vi "MSEncoder Case-4-IonGate.vi"(8 "error in (no error)":errorcluster, 9 "ParamValIn":variant, 11 "MSEncoder in":refnum<class "MSEncoder.lvclass">) -> (0 "error out":errorcluster, 3 "MSEncoder out":refnum<class "MSEncoder.lvclass">)   [LabVIEW 2018, in "MSEncoder.lvclass"]
uses:
  MSEncoder.lvclass
  Ctl/MSEditorParam ionGate.ctl
  MSEncoder.lvclass/MSEncoder.ctl
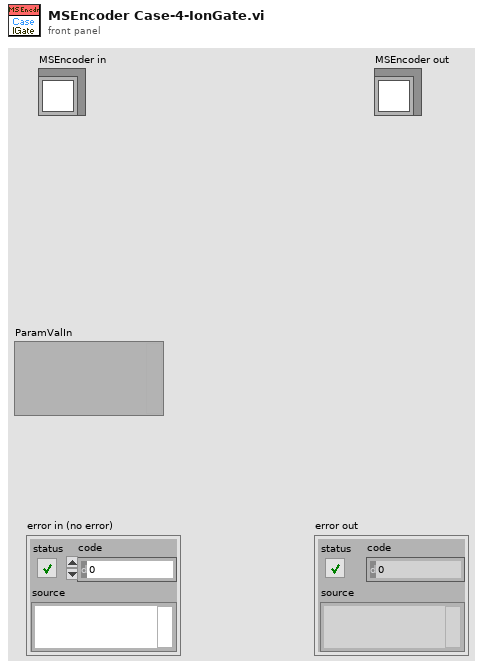
[diagram p1: front panel]
types:
  T1 = typedef "MSEditorParam ionGate.ctl" = cluster{"trialTime":ext, "TPH":ext, "enableAGC":bool}
  T2 = cluster{"Label":string, "dt":dbl, "Length":u32, "RefVolt":dbl, "mzTable":cluster{"t":dbl[], "mz":dbl[], "beta":dbl[]}}[]
  T3 = cluster{"Label":string, "dt":dbl, "Length":u32, "RefVolt":dbl, "mzTable":cluster{"t":dbl[], "mz":dbl[], "beta":dbl[]}}
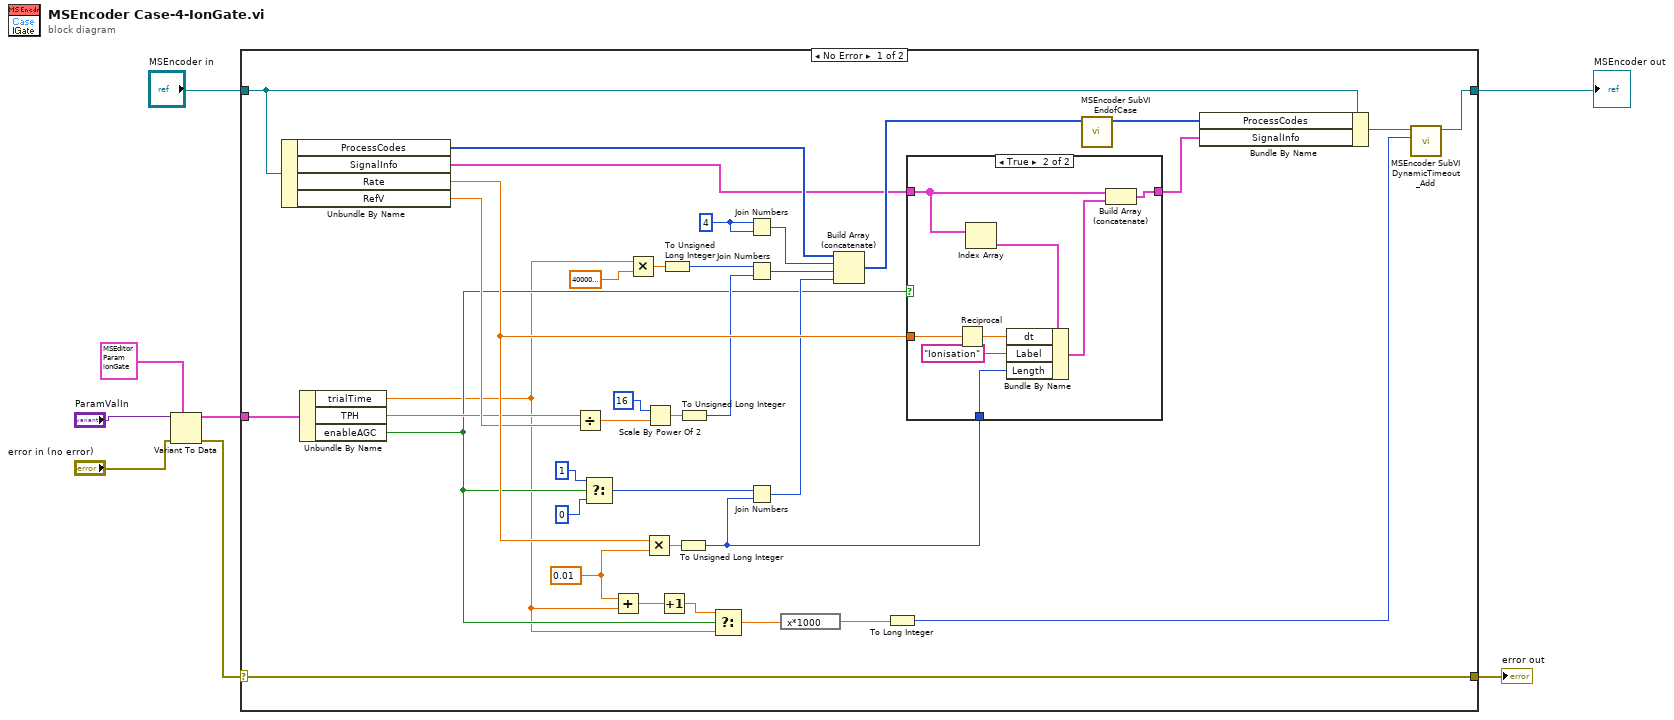
[diagram p0: block diagram]
diagram:
  n1 = Variant To Data(error in="error in (no error)", type=T1 {"trialTime"=0.1, "TPH"=1.0, "enableAGC"=FALSE} ("ParamValueType"), Variant="ParamValIn") -> (data=w2:T1, error out=w1:errorcluster)
  n2 = case shown="No Error" w1 {
    selector: w1 -> [w44 w56]
    tunnel: "MSEncoder in" -> [w43 w55]
    tunnel: [w44 w56] -> w8
    tunnel: [w17 w55] -> w6
    tunnel: w2 -> [w20 _]
    frame No Error {
      w11 = 0.01 ("y")
      w36 = u32 4
      n3 = Unbundle By Name(w43) -> ("ProcessCodes"=w45:u64[], "SignalInfo"=w15:T2, "Rate"=w41:dbl, "RefV"=w39:dbl)
      n4 = Unbundle By Name(w20) -> ("trialTime"=w10:ext, "TPH"=w21:ext, "enableAGC"=w16:bool)
      n5 = Divide(x=w21, y=w39) -> (x/y=w28:ext)
      n6 = Select(t=u32 1 ("n"), s=w16, f=u32 0 ("n")) -> (s? t:f=w23:u32)
      n7 = Add(x=w11, y=w10) -> (x+y=w12:ext)
      n8 = Multiply(x=w10, y=40000000.0) -> (x*y=w33:ext)
      n9 = Multiply(x=w41, y=w11) -> (x*y=w27:dbl)
      n10 = Scale By Power Of 2(n=i16 16, x=w28) -> (x*2^n=w37:ext)
      n11 = Increment(x=w12) -> (x+1=w9:ext)
      n12 = To Unsigned Long Integer(number=w33) -> (unsigned 32bit integer=w29:u32)
      n13 = To Unsigned Long Integer(number=w27) -> (unsigned 32bit integer=w24:u32)
      n14 = To Unsigned Long Integer(number=w37) -> (unsigned 32bit integer=w32:u32)
      n15 = Select(t=w9, s=w16, f=w10) -> (s? t:f=w14:ext)
      n16 = Join Numbers(hi=w36, lo=w36) -> ((hi.lo)=w35:u64)
      n17 = Join Numbers(hi=w29, lo=w32) -> ((hi.lo)=w31:u64)
      n18 = Join Numbers(hi=w23, lo=w24) -> ((hi.lo)=w30:u64)
      n19 = expression code="x*1000"(w14) -> (w13:ext)
      n20 = Build Array (concatenate)(w45, w35, w31, w30) -> (w22:u64[])
      n21 = To Long Integer(number=w13) -> (32bit integer=w19:i32)
      n22 = case shown="True" w16 {
        tunnel: w41 -> [_ w54]
        tunnel: [w46 w53] -> w40
        tunnel: w24 -> [_ w48]
        tunnel: w15 -> [w46 w47]
        frame False {
        }
        frame True {
          n23 = Reciprocal(x=w54) -> (1/x=w49:dbl)
          n24 = Index Array(array=w47) -> (element=w52:T3)  [unwired: 1 in]
          n25 = Bundle By Name(cluster=w52, "dt"=w49, "Label"="Ionisation", "Length"=w48) -> (w50:T3)
          n26 = Build Array (concatenate)(w47, w50) -> (w53:T2)
        }
      }
      n27 = call "MSEncoder SubVI EndofCase.vi"("Case codes"=w22) -> ("Case codes with end"=w42:u64[])  [unwired: 9 in, 1 out]
      n28 = Bundle By Name(cluster=w43, "ProcessCodes"=w42, "SignalInfo"=w40) -> (w18:refnum<class "MSEncoder.lvclass">)
      n29 = call "MSEncoder SubVI DynamicTimeout_Add.vi"("Timeout_ms"=w19, "MSEncoder"=w18) -> ("MSEncoder"=w17:refnum<class "MSEncoder.lvclass">)  [unwired: 8 in, 1 out]
    }
    frame Error {
    }
  }
  "error out" <- w8
  "MSEncoder out" <- w6
